vi "Initialize Attributes.vi"(8 "error in (no error)":errorcluster, 10 "Attribute Data":variant, 11 "CS++Motor in":refnum<class "CS++Motor.lvclass">) -> (0 "error out":errorcluster, 2 "Found?":bool, 3 "CS++Motor out":refnum<class "CS++Motor.lvclass">)   [LabVIEW 2015, in "CS++Motor.lvlib" / "CS++Motor.lvclass"]
doc: "Initialize object attribute.\n\nUnique resources should be allocated elsewhere!"
uses:
  CS++Motor.lvclass
  PV-Enum-n.ctl
  CSPP_Core/Classes/CS++ProcessVariables/ProcessVariable/PV.lvclass
  CSPP_Core/Actors/CS++BaseActor/CS++BaseActor.lvclass/CS++BaseActor.ctl
  CSPP_Core/Classes/CS++ProcessVariables/ProcessVariable/PV.lvclass/PV.ctl
  CS++Motor.lvclass/CS++Motor.ctl
  CSPP_Core/Classes/CS++ProcessVariables/ProcessVariable/Write PV URL.vi
  CSPP_Core/Classes/CS++ProcessVariables/ProcessVariable/Write Type Descriptor.vi
  <vilib>/Utility/error.llb/Error Cluster From Error Code.vi
  CSPP_Core/Actors/CS++DeviceActor/CS++DeviceActor.lvclass
  CSPP_Core/Classes/CS++BaseClasses/Factory/CS++Factory.lvclass
  CSPP_Core/Actors/CS++BaseActor/CS++BaseActor.lvclass
  CSPP_Core/Libraries/Utilities/CS++Utilities.lvlib
  CSPP_Core/Classes/CS++ProcessVariables/CS++ProcessVariables.lvlib
panel:
  in  "PV-Enum-n":T1
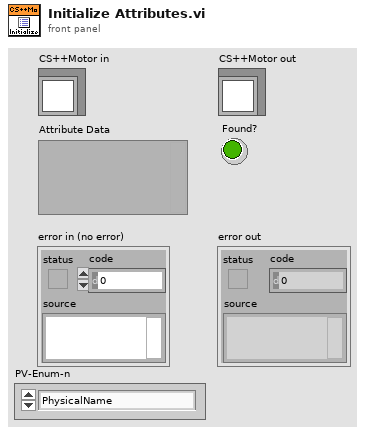
[diagram p1: front panel]
types:
  T1 = typedef "CS++Motor.lvlib/CS++Motor.lvclass/PV-Enum-n.ctl" = enum16{"PhysicalName", "unit", "SetPosition", "RawSetPosition", "StartVelocity", "StopVelocity", "Acceleration", "RangeMin", "RangeMax", "Scaling", "LogicalPositionArray"}
  T2 = cluster{"LogicalName":string, "PhysicalName":string, "unit":string, "Scaling":dbl, "SetPosition":dbl, "RawSetPosition":dbl, "StartVelocity":dbl, "StopVelocity":dbl, "Acceleration":dbl, "RangeMin":dbl, "RangeMax":dbl, "LogicalPos-Array":cluster{"LogicalPosition":string, "SetPosition":dbl}[]}
  T3 = cluster{"LogicalName":string, "PhysicalName":string, "unit":string, "Scaling":dbl, "SetPosition":dbl, "RawSetPosition":dbl, "StartVelocity":dbl, "StopVelocity":dbl, "Acceleration":dbl, "RangeMin":dbl, "RangeMax":dbl, "LogicalPos-Array":cluster{"LogicalPosition":string, "SetPosition":dbl}[]}[]
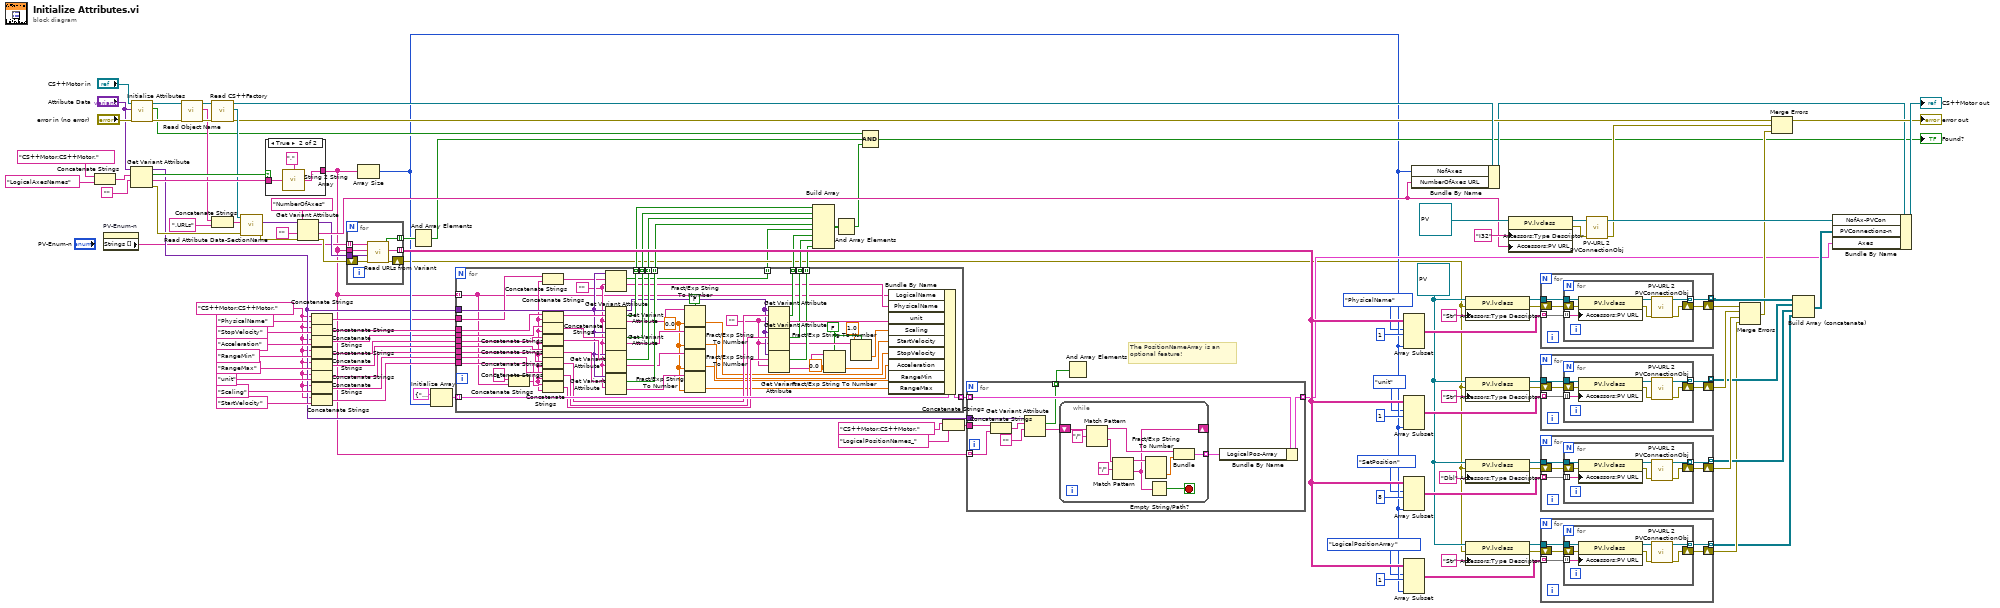
[diagram p0: block diagram]
diagram:
  w10 = "CS++Motor:CS++Motor."
  w16 = refnum<class "PV.lvclass"> refnum ("CS++ProcessVariables.lvlib:PV.lvclass")
  # "The PositionNameArray is an\noptional feature!"
  n1 = Concatenate Strings("CS++Motor:CS++Motor.", "LogicalAxesNames" ("string")) -> (w108:string)
  n2 = property on="PV-Enum-n" class="Enum (strict)"() -> ("Strings []"=w2:string[])  [unwired: 2 in, 2 out]
  n3 = Get Variant Attribute(Variant="Attribute Data", name=w108, default value (empty Variant)="") -> (duplicate Variant=w13:variant, found=w111:bool, value=w110:string, error out=w95:errorcluster)  [unwired: 1 in]
  n4 = call-parent "Initialize Attributes.vi"("error in (no error)"="error in (no error)", "Attribute Data"="Attribute Data", "CS++DeviceActor in"="CS++Motor in") -> ("error out"=w98:errorcluster, "Found?"=w59:bool, "CS++DeviceActor out"=w97:refnum<class "CS++Motor.lvclass">)  [unwired: 6 in]
  n5 = call "Read Object Name.vi"("error in (no error)"=w98, "CS++BaseActor in"=w97) -> ("error out"=w113:errorcluster, "Object Name"=w103:string, "CS++BaseActor out"=w114:refnum<class "CS++Motor.lvclass">)  [unwired: 7 in]
  n6 = call "Read CS++Factory.vi"("error in (no error)"=w113, "CS++BaseActor in"=w114) -> ("error out"=w70:errorcluster, "CS++Factory"=w102:refnum<class "CS++Factory.lvclass">, "CS++BaseActor out"=w94:refnum<class "CS++Motor.lvclass">)  [unwired: 7 in]
  n7 = Concatenate Strings(w103, ".URLs" ("string")) -> (w101:string)
  n8 = call-dynamic "Read Attribute Data-SectionName.vi"("error in (no error)"=w95, "Object Name"=w101, "CS++Factory in"=w102) -> ("error out"=w100:errorcluster, "Attribute Data"=w99:variant)  [unwired: 6 in, 1 out]
  n9 = case shown="True" w111 {
    tunnel: w110 -> [_ w119]
    tunnel: [_ w118] -> w1
    frame False {
    }
    frame True {
      n10 = call "String 2 String Array.vi"("String"=w119, "Delimiter (\",\")"="," ("Delimiter (\",\")")) -> ("Substrings"=w118:string[])
    }
  }
  n11 = Get Variant Attribute(Variant=w99, name="NumberOfAxes" ("string"), default value (empty Variant)="", error in=w100) -> (duplicate Variant=w7:variant, value=w64:string, error out=w92:errorcluster)  [unwired: 1 out]
  n12 = Concatenate Strings(w10, "PhysicalName") -> (w9:string)
  n13 = Concatenate Strings(w10, "StopVelocity") -> (w31:string)
  n14 = Concatenate Strings(w10, "Acceleration") -> (w12:string)
  n15 = Concatenate Strings(w10, "RangeMin") -> (w30:string)
  n16 = Concatenate Strings(w10, "RangeMax") -> (w29:string)
  n17 = Concatenate Strings(w10, "unit") -> (w28:string)
  n18 = Concatenate Strings(w10, "Scaling") -> (w27:string)
  n19 = Concatenate Strings(w10, "StartVelocity") -> (w26:string)
  n20 = for {
    tunnel: w2 -> [w120] mode=indexing
    tunnel: [w126] -> w61 mode=indexing
    tunnel: w7 -> [w124]
    tunnel: w1 -> [w123]
    tunnel: [w122] -> w41 mode=indexing
    shift-right: [w125] -> w14
    shift-left: w92 -> [w121]
    n21 = call "Read URLs from Variant.vi"("Error In"=w121, "URL Section Data"=w124, "Channel Names"=w123, "URL Prefix"=w120) -> ("Error Out"=w125:errorcluster, "URLs"=w122:string[], "Found?"=w126:bool)  [unwired: 5 in]
  }
  n22 = Array Size(array=w1) -> (size(s)=w15:i32)
  n23 = And Array Elements(Boolean array=w61) -> (logical AND=w60:bool)
  n24 = Initialize Array(T2 {"LogicalName"="", "PhysicalName"="", "unit"="", "Scaling"=0.0, "SetPosition"=0.0, "RawSetPosition"=0.0, "StartVelocity"=0.0, "StopVelocity"=0.0, "Acceleration"=0.0, "RangeMin"=0.0, "RangeMax"=0.0, "LogicalPos-Array"=[]} ("Cluster"), w15) -> (w43:T3)
  n25 = for {
    tunnel: w43 -> [w178] mode=indexing
    tunnel: [w177] -> w42 mode=indexing
    tunnel: w13 -> [w153]
    tunnel: [w175] -> w35 mode=indexing
    tunnel: [w174] -> w34 mode=indexing
    tunnel: [w173] -> w33 mode=indexing
    tunnel: [w172] -> w39 mode=indexing
    tunnel: [w171] -> w38 mode=indexing
    tunnel: [w170] -> w37 mode=indexing
    tunnel: [w169] -> w36 mode=indexing
    tunnel: w31 -> [w168]
    tunnel: w12 -> [w166]
    tunnel: w30 -> [w165]
    tunnel: w29 -> [w164]
    tunnel: w28 -> [w163]
    tunnel: w27 -> [w162]
    tunnel: w26 -> [w161]
    tunnel: w1 -> [w127] mode=indexing
    tunnel: w9 -> [w151]
    tunnel: [w148] -> w8 mode=indexing
    w131 = FALSE ("use system decimal point (T)")
    w138 = FALSE ("use system decimal point (T)")
    w136 = 0.0 ("default (0 DBL)")
    w137 = ""
    w130 = ""
    n26 = Concatenate Strings("_" ("string"), w127) -> (w149:string)
    n27 = Concatenate Strings(w151, w149) -> (w150:string)
    n28 = Concatenate Strings(w168, w149) -> (w160:string)
    n29 = Concatenate Strings(w166, w149) -> (w159:string)
    n30 = Concatenate Strings(w165, w149) -> (w158:string)
    n31 = Concatenate Strings(w164, w149) -> (w157:string)
    n32 = Concatenate Strings(w163, w149) -> (w156:string)
    n33 = Concatenate Strings(w162, w149) -> (w155:string)
    n34 = Concatenate Strings(w161, w149) -> (w154:string)
    n35 = Get Variant Attribute(Variant=w153, name=w150, default value (empty Variant)=w137) -> (found=w148:bool, value=w152:string)  [unwired: 1 in, 2 out]
    n36 = Get Variant Attribute(Variant=w153, name=w160, default value (empty Variant)=w137) -> (duplicate Variant=w139:variant, found=w172:bool, value=w147:string)  [unwired: 1 in, 1 out]
    n37 = Get Variant Attribute(Variant=w153, name=w159, default value (empty Variant)=w137) -> (found=w171:bool, value=w145:string)  [unwired: 1 in, 2 out]
    n38 = Get Variant Attribute(Variant=w153, name=w158, default value (empty Variant)=w137) -> (found=w170:bool, value=w143:string)  [unwired: 1 in, 2 out]
    n39 = Get Variant Attribute(Variant=w153, name=w157, default value (empty Variant)=w137) -> (found=w169:bool, value=w141:string)  [unwired: 1 in, 2 out]
    n40 = Fract/Exp String To Number(use system decimal point (T)=w138, string=w147, default (0 dbl)=w136) -> (number=w146:dbl)  [unwired: 1 in, 1 out]
    n41 = Fract/Exp String To Number(use system decimal point (T)=w138, string=w145, default (0 dbl)=w136) -> (number=w144:dbl)  [unwired: 1 in, 1 out]
    n42 = Fract/Exp String To Number(use system decimal point (T)=w138, string=w143, default (0 dbl)=w136) -> (number=w142:dbl)  [unwired: 1 in, 1 out]
    n43 = Fract/Exp String To Number(use system decimal point (T)=w138, string=w141, default (0 dbl)=w136) -> (number=w140:dbl)  [unwired: 1 in, 1 out]
    n44 = Get Variant Attribute(Variant=w139, name=w156, default value (empty Variant)=w130) -> (found=w175:bool, value=w176:string)  [unwired: 1 in, 2 out]
    n45 = Get Variant Attribute(Variant=w139, name=w155, default value (empty Variant)=w130) -> (found=w174:bool, value=w135:string)  [unwired: 1 in, 2 out]
    n46 = Get Variant Attribute(Variant=w139, name=w154, default value (empty Variant)=w130) -> (found=w173:bool, value=w133:string)  [unwired: 1 in, 2 out]
    n47 = Fract/Exp String To Number(use system decimal point (T)=w131, string=w133, default (0 dbl)=0.0 ("default (0 DBL)")) -> (number=w132:dbl)  [unwired: 1 in, 1 out]
    n48 = Fract/Exp String To Number(use system decimal point (T)=w131, string=w135, default (0 dbl)=1.0 ("default (0 DBL)")) -> (number=w134:dbl)  [unwired: 1 in, 1 out]
    n49 = Bundle By Name(cluster=w178, "LogicalName"=w127, "PhysicalName"=w152, "unit"=w176, "Scaling"=w134, "StartVelocity"=w132, "StopVelocity"=w146, "Acceleration"=w144, "RangeMin"=w142, "RangeMax"=w140) -> (w177:T2)
  }
  n50 = Build Array(w39, w38, w37, w36, w8, w35, w34, w33) -> (w32:bool[][])
  n51 = And Array Elements(Boolean array=w32) -> (logical AND=w40:bool)
  n52 = Compound Arithmetic op=AND(w59, w60, w40) -> (→"Found?":bool)
  n53 = Concatenate Strings("CS++Motor:CS++Motor.", "LogicalPositionNames_" ("string")) -> (w53:string)
  n54 = for {
    tunnel: w42 -> [w188] mode=indexing
    tunnel: [w187] -> w17 mode=indexing
    tunnel: w13 -> [w186]
    tunnel: w53 -> [w183]
    tunnel: [w181] -> w52 mode=indexing
    tunnel: w1 -> [w179] mode=indexing
    n55 = Concatenate Strings(w183, w179) -> (w184:string)
    n56 = Get Variant Attribute(Variant=w186, name=w184, default value (empty Variant)="") -> (found=w181:bool, value=w182:string)  [unwired: 1 in, 2 out]
    n57 = while {
      tunnel: [w195] -> w180 mode=indexing
      shift-right: [w190] -> _
      shift-left: w182 -> [w198]
      stop <- w189 stop-if-true
      n58 = Match Pattern(string=w198, regular expression="/") -> (before substring=w196:string, after substring=w193:string)  [unwired: 1 in, 2 out]
      n59 = Match Pattern(string=w193, regular expression="/") -> (before substring=w191:string, after substring=w190:string)  [unwired: 1 in, 2 out]
      n60 = Fract/Exp String To Number(string=w191) -> (number=w192:dbl)  [unwired: 3 in, 1 out]
      n61 = Empty String/Path?(string/path=w190) -> (empty?=w189:bool)
      n62 = Bundle(w196, w192) -> (w195:cluster{string, dbl})  [unwired: 1 in]
    }
    n63 = Bundle By Name(cluster=w188, "LogicalPos-Array"=w180) -> (w187:T2)
  }
  n64 = And Array Elements(Boolean array=w52) -> ()  [unwired: 1 out]
  n65 = Array Subset(array=w41, index (row)=PV-Enum-n."PhysicalName" ("PV-Enum-n"), length (row)=1 ("length"), length (col)=w15) -> (w91:string[][])  [unwired: 1 in]
  n66 = Array Subset(array=w41, index (row)=PV-Enum-n."unit" ("PV-Enum-n"), length (row)=1 ("length"), length (col)=w15) -> (w86:string[][])  [unwired: 1 in]
  n67 = Array Subset(array=w41, index (row)=PV-Enum-n."SetPosition" ("PV-Enum-n"), length (row)=8 ("length"), length (col)=w15) -> (w81:string[][])  [unwired: 1 in]
  n68 = Array Subset(array=w41, index (row)=PV-Enum-n."LogicalPositionArray" ("PV-Enum-n"), length (row)=1 ("length"), length (col)=w15) -> (w44:string[][])  [unwired: 1 in]
  n69 = Bundle By Name(cluster=w94, "NofAxes"=w15, "NumberOfAxes URL"=w64) -> (w56:refnum<class "CS++Motor.lvclass">)
  n70 = property class="PV.lvclass"(reference=w16, error in=w14, "Accessors:Type Descriptor"="Str" ("Type Descriptor")) -> (reference out=w89:refnum<class "PV.lvclass">, error out=w88:errorcluster)
  n71 = property class="PV.lvclass"(reference=w16, error in=w14, "Accessors:Type Descriptor"="Str" ("Type Descriptor")) -> (reference out=w84:refnum<class "PV.lvclass">, error out=w83:errorcluster)
  n72 = property class="PV.lvclass"(reference=w16, error in=w14, "Accessors:Type Descriptor"="Dbl" ("Type Descriptor")) -> (reference out=w79:refnum<class "PV.lvclass">, error out=w78:errorcluster)
  n73 = property class="PV.lvclass"(reference=w16, error in=w14, "Accessors:Type Descriptor"="Str" ("Type Descriptor")) -> (reference out=w49:refnum<class "PV.lvclass">, error out=w48:errorcluster)
  n74 = property class="PV.lvclass"(reference=refnum<class "PV.lvclass"> refnum ("CS++ProcessVariables.lvlib:PV.lvclass"), "Accessors:Type Descriptor"="I32" ("Type Descriptor"), "Accessors:PV URL"=w64) -> (reference out=w65:refnum<class "PV.lvclass">, error out=w66:errorcluster)  [unwired: 1 in]
  n75 = for {
    tunnel: w89 -> [w203]
    tunnel: w91 -> [w202] mode=indexing
    tunnel: [w201] -> w73 mode=indexing
    shift-right: [w200] -> w76
    shift-left: w88 -> [w199]
    n76 = for {
      tunnel: w203 -> [w209]
      tunnel: w202 -> [w208] mode=indexing
      tunnel: [w207] -> w201 mode=indexing
      shift-right: [w206] -> w200
      shift-left: w199 -> [w204]
      n77 = property class="PV.lvclass"(reference=w209, error in=w204, "Accessors:PV URL"=w208) -> (reference out=w210:refnum<class "PV.lvclass">, error out=w205:errorcluster)
      n78 = call "PV-URL 2 PVConnectionObj.vi"("Error In"=w205, "PV"=w210) -> ("Error Out"=w206:errorcluster, "PVConnection"=w207:refnum<class "PVConnection.lvclass">)  [unwired: 7 in, 1 out]
    }
  }
  n79 = for {
    tunnel: w84 -> [w215]
    tunnel: w86 -> [w214] mode=indexing
    tunnel: [w213] -> w72 mode=indexing
    shift-right: [w212] -> w75
    shift-left: w83 -> [w211]
    n80 = for {
      tunnel: w215 -> [w221]
      tunnel: w214 -> [w220] mode=indexing
      tunnel: [w219] -> w213 mode=indexing
      shift-right: [w218] -> w212
      shift-left: w211 -> [w216]
      n81 = property class="PV.lvclass"(reference=w221, error in=w216, "Accessors:PV URL"=w220) -> (reference out=w222:refnum<class "PV.lvclass">, error out=w217:errorcluster)
      n82 = call "PV-URL 2 PVConnectionObj.vi"("Error In"=w217, "PV"=w222) -> ("Error Out"=w218:errorcluster, "PVConnection"=w219:refnum<class "PVConnection.lvclass">)  [unwired: 7 in, 1 out]
    }
  }
  n83 = for {
    tunnel: w79 -> [w227]
    tunnel: w81 -> [w226] mode=indexing
    tunnel: [w225] -> w71 mode=indexing
    shift-right: [w224] -> w74
    shift-left: w78 -> [w223]
    n84 = for {
      tunnel: w227 -> [w233]
      tunnel: w226 -> [w232] mode=indexing
      tunnel: [w231] -> w225 mode=indexing
      shift-right: [w230] -> w224
      shift-left: w223 -> [w228]
      n85 = property class="PV.lvclass"(reference=w233, error in=w228, "Accessors:PV URL"=w232) -> (reference out=w234:refnum<class "PV.lvclass">, error out=w229:errorcluster)
      n86 = call "PV-URL 2 PVConnectionObj.vi"("Error In"=w229, "PV"=w234) -> ("Error Out"=w230:errorcluster, "PVConnection"=w231:refnum<class "PVConnection.lvclass">)  [unwired: 7 in, 1 out]
    }
  }
  n87 = for {
    tunnel: w49 -> [w239]
    tunnel: w44 -> [w238] mode=indexing
    tunnel: [w237] -> w45 mode=indexing
    shift-right: [w236] -> w46
    shift-left: w48 -> [w235]
    n88 = for {
      tunnel: w239 -> [w245]
      tunnel: w238 -> [w244] mode=indexing
      tunnel: [w243] -> w237 mode=indexing
      shift-right: [w242] -> w236
      shift-left: w235 -> [w240]
      n89 = property class="PV.lvclass"(reference=w245, error in=w240, "Accessors:PV URL"=w244) -> (reference out=w246:refnum<class "PV.lvclass">, error out=w241:errorcluster)
      n90 = call "PV-URL 2 PVConnectionObj.vi"("Error In"=w241, "PV"=w246) -> ("Error Out"=w242:errorcluster, "PVConnection"=w243:refnum<class "PVConnection.lvclass">)  [unwired: 7 in, 1 out]
    }
  }
  n91 = call "PV-URL 2 PVConnectionObj.vi"("Error In"=w66, "PV"=w65) -> ("Error Out"=w57:errorcluster, "PVConnection"=w63:refnum<class "PVConnection.lvclass">)  [unwired: 7 in, 1 out]
  n92 = Merge Errors(w76, w75, w74, w46) -> (w58:errorcluster)
  n93 = Merge Errors(w70, w57, w58) -> (→"error out":errorcluster)
  n94 = Build Array (concatenate)(w73, w72, w71, w45) -> (w62:refnum<class "PVConnection.lvclass">[][])
  n95 = Bundle By Name(cluster=w56, "NofAx-PVCon"=w63, "PVConnections-n"=w62, "Axes"=w17) -> (→"CS++Motor out":refnum<class "CS++Motor.lvclass">)
